vi "Initialise GPIB Controller.vi"(4 "error in (no error)":errorcluster, 6 "Address":u32=1, 7 "VISA resource name":refnum<visa-resource-name>) -> (0 "error out":errorcluster, 3 "VISA resource name out":refnum<visa-resource-name>)   [LabVIEW 2015]
doc: "Setup the VISA link to the Prologix GPIB-USB Controller."
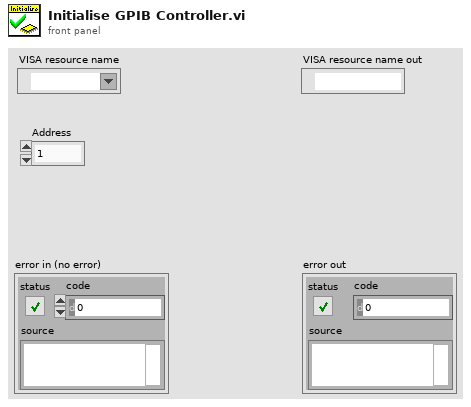
[diagram p1: front panel]
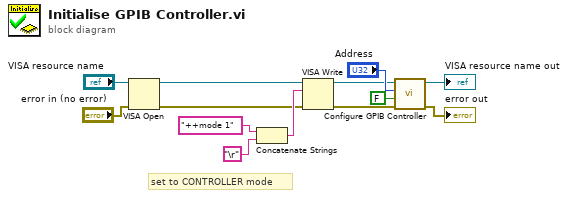
[diagram p0: block diagram]
diagram:
  # "set to CONTROLLER mode"
  n1 = VISA Open(error in (no error)="error in (no error)", VISA resource name="VISA resource name") -> (VISA resource name=w5:refnum<visa-resource-name>, error out=w4:errorcluster)  [unwired: 3 in]
  n2 = Concatenate Strings("++mode 1" ("write buffer"), "\r") -> (w10:string)
  n3 = VISA Write(VISA resource name=w5, write buffer=w10, error in (no error)=w4) -> (VISA resource name out=w3:refnum<visa-resource-name>, error out=w2:errorcluster)  [unwired: 1 out]
  n4 = call "Configure GPIB Controller.vi"("error in (no error)"=w2, "Read-after-Write?"=FALSE, "Address"="Address", "VISA Refnum in"=w3) -> ("error out"=→"error out":errorcluster, "VISA Refnum out"=→"VISA resource name out":refnum<visa-resource-name>)  [unwired: 6 in]
